vi "Driver - DTACQ - Send Synchronous Message (Termex Acknowledged).vi"(8 "error in":errorcluster, 10 "Message to Send":string, 11 "DTACQ Connection Data In":T1={"Description"="", "Address"="", "Port"=0, "timeout (ms)"=5000, "Termination Character"="\n", "TCP Connection Reference"=refnum, "Open Connection"=FALSE}) -> (0 "error out":errorcluster, 1 "Timed Out":bool=TRUE, 2 "Message Acknowledged":bool, 3 "DTACQ Connection Data Out":T1={"Description"="", "Address"="", "Port"=0, "timeout (ms)"=5000, "Termination Character"="\n", "TCP Connection Reference"=refnum, "Open Connection"=FALSE})   [LabVIEW 2017, in "Communications Library.lvlib"]
doc: "Writes a string to a DTACQ device using TCP and reads the response.\n\nOpens the TCP connection, if it is not already open."
uses:
  Communications Library.lvlib
  Typedefs/DTACQ Connection Data--Cluster.ctl
  Debug - Lower Level - Logging Tool.vi
  Error 5102 - DTACQ unit replied with an error--const.vi
  <vilib>/Utility/error.llb/Error Cluster From Error Code.vi
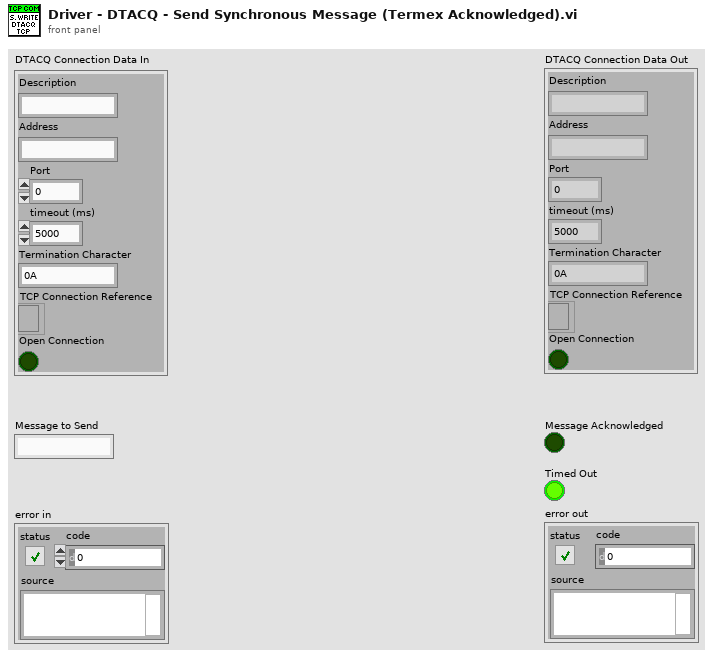
[diagram p1: front panel]
types:
  T1 = typedef "Communications Library.lvlib/DTACQ Connection Data--Cluster.ctl" = cluster{"Description":string, "Address":string, "Port":u16, "timeout (ms)":i32, "Termination Character":string, "TCP Connection Reference":refnum<k5>, "Open Connection":bool}
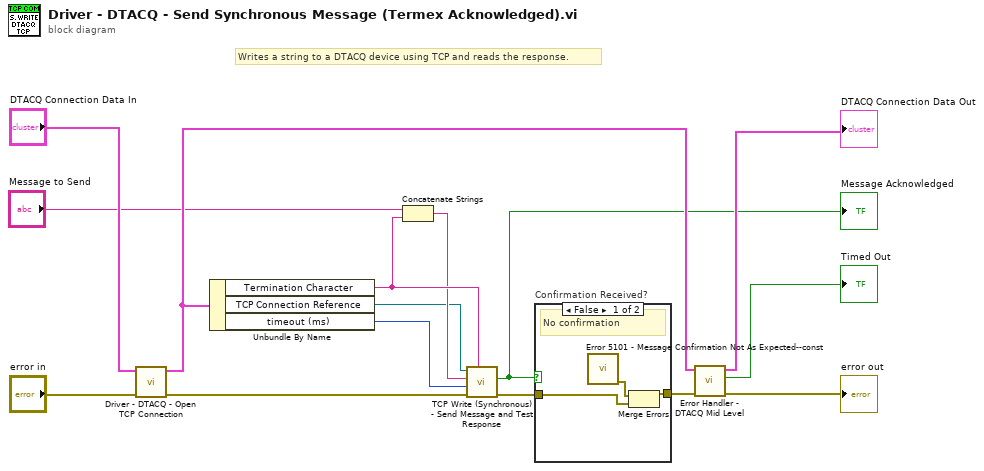
[diagram p0: block diagram]
diagram:
  # "Writes a string to a DTACQ device using TCP and reads the response."
  n1 = call "Driver - DTACQ - Open TCP Connection.vi"("error in"="error in", "DTACQ Connection Data In"="DTACQ Connection Data In") -> ("error out"=w9:errorcluster, "DTACQ Connection Data Out"=w11:T1)  [unwired: 8 in]
  n2 = Unbundle By Name(w11) -> ("Termination Character"=w7:string, "TCP Connection Reference"=w5:refnum<k5>, "timeout (ms)"=w4:i32)
  n3 = Concatenate Strings("Message to Send", w7) -> (w6:string)
  n4 = call "TCP Write (Synchronous) - Send Message and Test Response.vi"("Expected Response"=w7, "error in"=w9, "Timeout (ms)"=w4, "Data to Write"=w6, "TCP Network Connecion In"=w5) -> ("error out"=w2:errorcluster, "Valid Response"=w3:bool)  [unwired: 3 in, 2 out]
  "Message Acknowledged" <- w3
  n5 = case "Confirmation Received?" shown="False" w3 {
    tunnel: w2 -> [w16 w19]
    tunnel: [w18 w19] -> w1
    frame False {
      # "No confirmation"
      n6 = call "Error 5101 - Message Confirmation Not As Expected--const.vi"() -> ("error out"=w17:errorcluster)  [unwired: 11 in]
      n7 = Merge Errors(w17, w16) -> (w18:errorcluster)
    }
    frame True {
      # "Yes, termination\ncharacter confirmed\nmessage receipt."
    }
  }
  n8 = call "Error Handler - DTACQ Mid Level.vi"("error in"=w1, "DTACQ Connection Data In"=w11) -> ("error out"=→"error out":errorcluster, "Timed Out"=→"Timed Out":bool, "DTACQ Connection Data Out"=→"DTACQ Connection Data Out":T1)  [unwired: 7 in]
